vi "Accumulcate Execution Time.vi"(10 "Result":T1={"Name"="", "Message"="", "Description"="", "Status"=enum."Passed", "Result Type"=enum."Test Suite", "Execution Time"=0.0}, 11 "Result Model in":refnum<class "Result Model.lvclass">) -> ()   [LabVIEW 2020, in "Result Model.lvclass"]
uses:
  Result Model.lvclass
  Core/Result/Result.ctl
  Core/Result/Status.ctl
  Core/Result/Type.ctl
  Result Model.lvclass/Result Model.ctl
  <vilib>/Utility/miscctls.llb/LVMapReplaceAction.ctl
  Core/Result/Result.lvlib
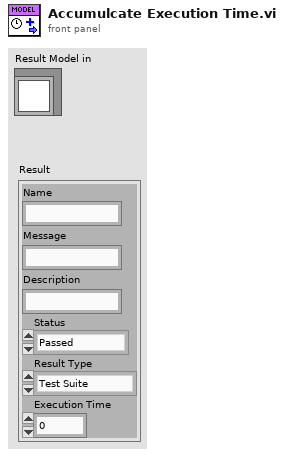
[diagram p1: front panel]
types:
  T1 = typedef "Result.lvlib/Result.ctl" = cluster{"Name":string, "Message":string, "Description":string, "Status":T2, "Result Type":T3, "Execution Time":dbl}
  T2 = typedef "Result.lvlib/Status.ctl" = enum16{"", "Passed", "Failed", "Error", "Skipped", "Setup Error", "Broken", "Teardown Error"}
  T3 = typedef "Result.lvlib/Type.ctl" = enum16{"Test Case", "Test Suite", "Test Run", "Pass", "Fail", "Skip", "Pass if", "Fail if", "Pass if Error", "Fail if Error", "Pass if Equal", "Fail if Equal"}
  T4 = typedef "LVMapReplaceAction.ctl" = enum32{"Modify Entry only if found", "Add or Modify Entry", "Delete Entry"}
  T5 = typedef "Result Model.lvclass/Model State.ctl" = cluster{"Run Queue":set{string}, "Test Statuses":map{string, T2}, "Execution Time":map{string, dbl}, "Assertions":map{string, cluster{"Result Type":T3, "Status":T2, "Message":string, "Description":string}[]}}
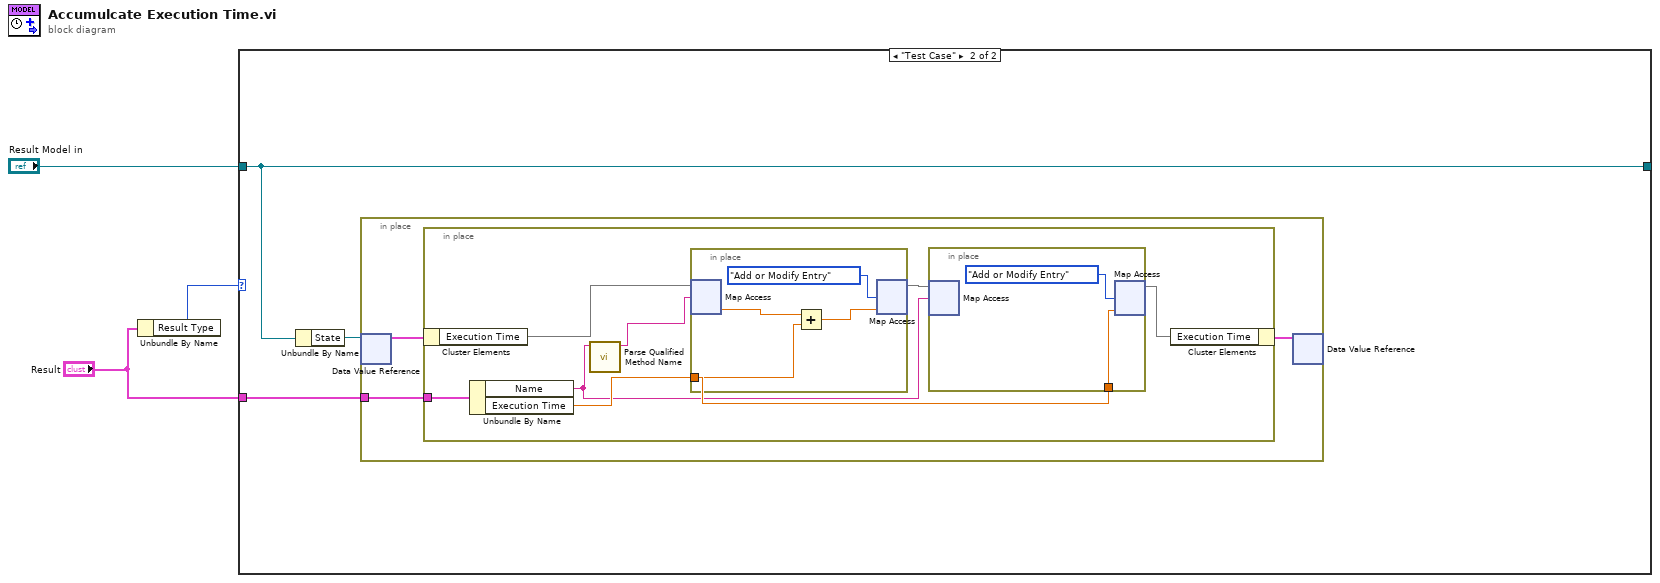
[diagram p0: block diagram]
diagram:
  n1 = Unbundle By Name("Result") -> ("Result Type"=w1:T3)
  n2 = case shown="\"Test Case\"" w1 {
    tunnel: "Result" -> [_ w7]
    tunnel: "Result Model in" -> [w4 w6]
    tunnel: [w4 w6] -> _
    frame Default {
    }
    frame "Test Case" {
      n3 = Unbundle By Name(w6) -> ("State"=w5:refnum<data-value>)
      n4 = in-place {
        in-place-border: w7 -> [w10]
        n5 = in-place-dvr #1(w5) -> (w9:T5)  [unwired: 1 out]
        n6 = in-place {
          in-place-border: w10 -> [w16]
          n7 = in-place-cluster #2(w9) -> ("Execution Time"=w12:map{string, dbl})
          n8 = Unbundle By Name(w16) -> ("Name"=w14:string, "Execution Time"=w15:dbl)
          n9 = call "Parse Qualified Method Name.vi"("Case"=w14) -> ("Test Case Class Name"=w13:string)  [unwired: 9 in, 1 out]
          n10 = in-place {
            in-place-border: w15 -> [w21]
            n11 = in-place-map #3(w12, w13) -> (w20:dbl)  [unwired: 1 in, 1 out]
            n12 = Add(x=w20, y=w21) -> (x+y=w23:dbl)
            n13 = in-place-map #3(w23, LVMapReplaceAction."Add or Modify Entry" ("action")) -> (w17:map{string, dbl})  [unwired: 2 out]
          }
          n14 = in-place {
            in-place-border: w15 -> [w18]
            n15 = in-place-map #4(w17, w14) -> ()  [unwired: 1 in, 2 out]
            n16 = in-place-map #4(w18, LVMapReplaceAction."Add or Modify Entry" ("action")) -> (w11:map{string, dbl})  [unwired: 2 out]
          }
          n17 = in-place-cluster #2("Execution Time"=w11) -> (w8:T5)
        }
        n18 = in-place-dvr #1(w8) -> ()  [unwired: 2 out]
      }
    }
  }
